vi "XBEE Rx Serial Frame Processor.vi"(9 "RX Frame Queue":refnum<queue>, 11 "VISA Serial Port":refnum<visa-resource-name>) -> (0 "error out":errorcluster)   [LabVIEW 2017]
uses:
  WiFi API Frame.ctl
  WiFi API Frame Type.ctl
  stop button.vi
panel:
  in  "stop":bool
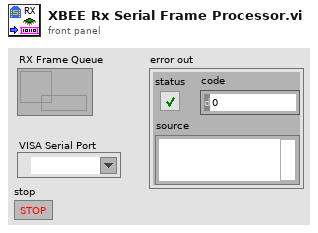
[diagram p1: front panel]
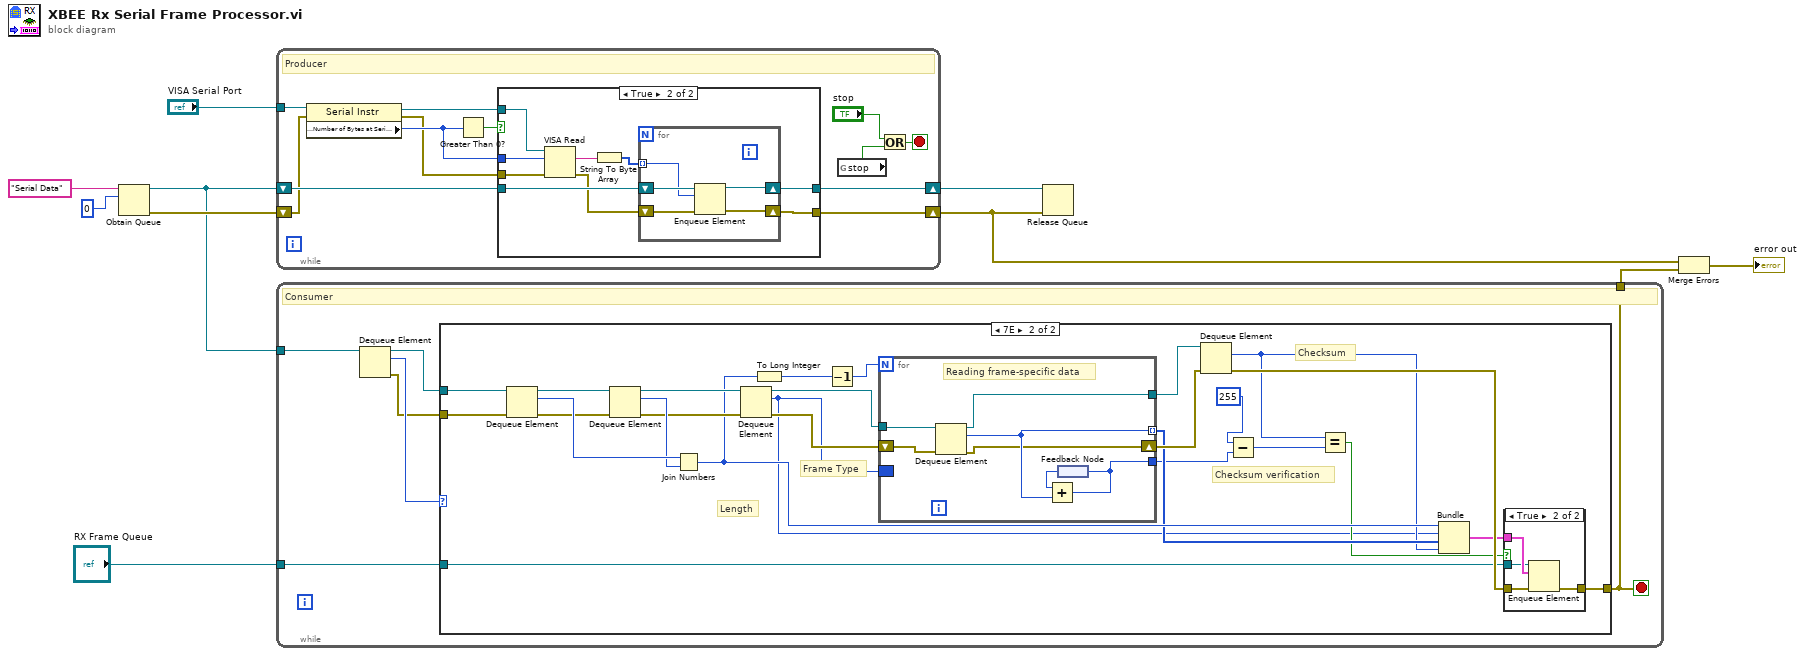
[diagram p0: block diagram]
diagram:
  n1 = Obtain Queue(name (unnamed)="Serial Data", element data type=u8 0) -> (queue out=w6:refnum<queue>, error out=w7:errorcluster)  [unwired: 3 in, 1 out]
  n2 = while {
    tunnel: "VISA Serial Port" -> [w22]
    shift-right: [w17] -> w5
    shift-left: w6 -> [w20]
    shift-right: [w14] -> w1
    shift-left: w7 -> [w16]
    stop <- w13 stop-if-true
    # "Producer"
    n3 = property class="Serial Instr"(reference=w22, error in=w16) -> (reference out=w19:refnum<visa-resource-name>, error out=w15:errorcluster, "Serial Settings:Number of Bytes at Serial Port"=w18:u32)
    n4 = Greater Than 0?(x=w18) -> (x > 0?=w21:bool)
    n5 = case shown="True" w21 {
      tunnel: w20 -> [w24 w28]
      tunnel: w19 -> [_ w33]
      tunnel: w18 -> [_ w32]
      tunnel: w15 -> [w23 w30]
      tunnel: [w24 w27] -> w17
      tunnel: [w23 w26] -> w14
      frame False {
      }
      frame True {
        n6 = VISA Read(VISA resource name=w33, byte count=w32, error in (no error)=w30) -> (read buffer=w31:string, error out=w25:errorcluster)  [unwired: 2 out]
        n7 = String To Byte Array(string=w31) -> (unsigned byte array=w29:u8[])
        n8 = for {
          tunnel: w29 -> [w37] mode=indexing
          shift-right: [w36] -> w27
          shift-left: w28 -> [w38]
          shift-right: [w35] -> w26
          shift-left: w25 -> [w34]
          n9 = Enqueue Element(queue=w38, element=w37, error in (no error)=w34) -> (queue out=w36:refnum<queue>, error out=w35:errorcluster)  [unwired: 1 in, 1 out]
        }
      }
    }
    n10 = global read "stop button.vi" "stop"() -> (w11:bool)
    n11 = Or(x="stop", y=w11) -> (x .or. y?=w13:bool)
  }
  n12 = while {
    tunnel: w6 -> [w44]
    tunnel: [w41] -> w4
    tunnel: "RX Frame Queue" -> [w40]
    stop <- w41 stop-if-true
    # "Consumer"
    n13 = Dequeue Element(queue=w44) -> (queue out=w39:refnum<queue>, element=w43:u8, error out=w42:errorcluster)  [unwired: 2 in, 1 out]
    n14 = case shown="7E" w43 {
      tunnel: w39 -> [_ w71]
      tunnel: w42 -> [w45 w60]
      tunnel: w40 -> [_ w52]
      tunnel: [w45 w54] -> w41
      frame 0, Default {
      }
      frame 126 {
        # "Checksum"
        # "Length"
        # "Checksum verification"
        # "Frame Type"
        n15 = Dequeue Element(queue=w71, error in (no error)=w60) -> (queue out=w70:refnum<queue>, element=w69:u8, error out=w61:errorcluster)  [unwired: 1 in, 1 out]
        n16 = Dequeue Element(queue=w70, error in (no error)=w61) -> (queue out=w67:refnum<queue>, element=w68:u8, error out=w62:errorcluster)  [unwired: 1 in, 1 out]
        n17 = Join Numbers(hi=w69, lo=w68) -> ((hi.lo)=w57:u16)
        n18 = Dequeue Element(queue=w67, error in (no error)=w62) -> (queue out=w66:refnum<queue>, element=w46:u8, error out=w63:errorcluster)  [unwired: 1 in, 1 out]
        n19 = To Long Integer(number=w57) -> (32bit integer=w64:i32)
        n20 = Decrement(x=w64) -> (x-1=w65:i32)
        n21 = for {
          N: w65 -> [_]
          tunnel: w66 -> [w83]
          tunnel: [w79] -> w56 mode=indexing
          tunnel: [w81] -> w59
          tunnel: [w80] -> w49
          shift-right: [w77] -> w58
          shift-left: w63 -> [w82]
          border: w46 -> [_]
          # "Reading frame-specific data"
          n22 = Dequeue Element(queue=w83, error in (no error)=w82) -> (queue out=w81:refnum<queue>, element=w79:u8, error out=w77:errorcluster)  [unwired: 1 in, 1 out]
          n23 = feedback #1() -> (w78:u8)
          n24 = Add(x=w78, y=w79) -> (x+y=w80:u8)
          n25 = feedback-in #1(w80) -> ()
        }
        n26 = Dequeue Element(queue=w59, error in (no error)=w58) -> (element=w48:u8, error out=w55:errorcluster)  [unwired: 1 in, 2 out]
        n27 = Subtract(x=u8 255, y=w49) -> (x-y=w47:u8)
        n28 = Equal?(x=w48, y=w47) -> (x = y?=w51:bool)
        n29 = Bundle(w57, w46, w56, w48) -> (w53:cluster{u16, u8, u8[], u8})  [unwired: 1 in]
        n30 = case shown="True" w51 {
          tunnel: w55 -> [w72 w76]
          tunnel: [w72 w75] -> w54
          tunnel: w53 -> [_ w74]
          tunnel: w52 -> [_ w73]
          frame False {
          }
          frame True {
            n31 = Enqueue Element(queue=w73, element=w74, error in (no error)=w76) -> (error out=w75:errorcluster)  [unwired: 1 in, 2 out]
          }
        }
      }
    }
  }
  n32 = Release Queue(queue=w5, error in (no error)=w1) -> ()  [unwired: 1 in, 3 out]
  n33 = Merge Errors(w1, w4) -> (→"error out":errorcluster)
